vi "公式发生改变存储 (子VI).vi"(6 "公式":cluster{"X^2":dbl, "X":dbl, "b":dbl}, 9 "量程下拉列表输入":refnum<vi>, 10 "测量模式下拉列表输入":refnum<vi>, 11 "参数":refnum<vi>) -> ()   [LabVIEW 2016, in "斯坦道总氮.lvlib"]
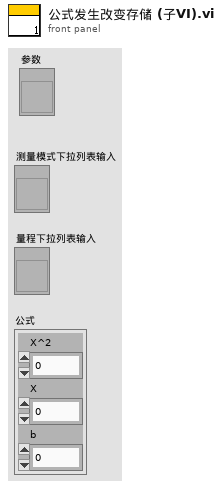
[diagram p1: front panel]
types:
  T1 = cluster{"时间标识":timestamp, "设备":string, "日志信息":string, "流程参数":string}
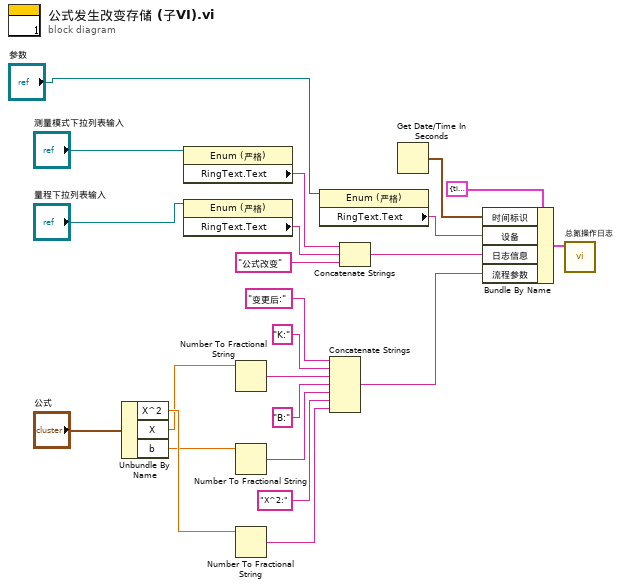
[diagram p0: block diagram]
diagram:
  n1 = Unbundle By Name("公式") -> ("X^2"=w19:dbl, "X"=w17:dbl, "b"=w18:dbl)
  n2 = property on="属性节点" class="Enum (严格)"(reference="测量模式下拉列表输入") -> ("RingText.Text"=w6:string)  [unwired: 1 in, 2 out]
  n3 = property on="属性节点" class="Enum (严格)"(reference="量程下拉列表输入") -> ("RingText.Text"=w7:string)  [unwired: 1 in, 2 out]
  n4 = Number To Fractional String(number=w17) -> (F-format string=w13:string)  [unwired: 3 in]
  n5 = Number To Fractional String(number=w18) -> (F-format string=w14:string)  [unwired: 3 in]
  n6 = Number To Fractional String(number=w19) -> (F-format string=w15:string)  [unwired: 3 in]
  n7 = property class="Enum (严格)"(reference="参数") -> ("RingText.Text"=w23:string)  [unwired: 1 in, 2 out]
  n8 = Concatenate Strings("变更后:" ("table输入"), "K:" ("字符串"), w13, "B:" ("字符串"), w14, "X^2:" ("字符串"), w15) -> (w2:string)
  n9 = Concatenate Strings(w6, w7, "公式改变" ("日志信息")) -> (w22:string)
  n10 = Get Date/Time In Seconds() -> (seconds since 1Jan1904=w3:timestamp)
  n11 = Bundle By Name(cluster=T1 {"时间标识"=timestamp(0 s since 1904-01-01), "设备"="", "日志信息"="", "流程参数"=""} ("data in"), "时间标识"=w3, "设备"=w23, "日志信息"=w22, "流程参数"=w2) -> (w4:T1)
  n12 = call "总氮操作日志.vi"("data in"=w4) -> ()  [unwired: 11 in]
